vi "uActor_Set_uErrClass(Conditional).vi"(10 "uErr":refnum<class "uErr.lvclass">, 11 "uActor in":refnum<class "uActor.lvclass">) -> (3 "uActor out":refnum<class "uActor.lvclass">)   [LabVIEW 2023, in "uFramework.lvlib" / "uActor.lvclass"]
doc: "Use at runtime to set the Error handling behavior of an actor. This method executes only if there is not uErr class behavior assigned already to this actor. If there is a preassigned error behavior assignment, then this method ignores the new output."
uses:
  uActor.lvclass
  uErr/uErr.lvclass
  uActor.lvclass/uActor.ctl
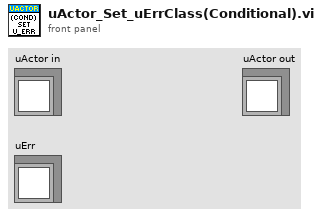
[diagram p1: front panel]
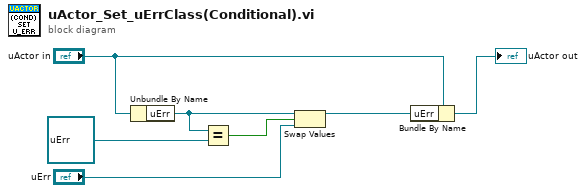
[diagram p0: block diagram]
diagram:
  n1 = Unbundle By Name("uActor in") -> ("uErr"=w1:refnum<class "uErr.lvclass">)
  n2 = Equal?(x=w1, y=refnum<class "uErr.lvclass"> refnum ("x")) -> (x = y?=w3:bool)
  n3 = Swap Values(12:w1, 13:w3, 14:"uErr") -> (1:w6:refnum<class "uErr.lvclass">)  [unwired: 1 out]
  n4 = Bundle By Name(cluster="uActor in", "uErr"=w6) -> (→"uActor out":refnum<class "uActor.lvclass">)
